vi "GetESN.vi"(9 "MEID":string, 10 "Data":string[][](array[string])=[["8986031490021881534", "460036161669975", "2A645416CB435F94", "8006A127", "460036161669975@mycdma.cn", "DB60264368A1D188", "18101891253", "A1000021A59070"], ["8986031490021881535", "460036161669976", "32FA5764D69C76BE", "80FAE4E6", "460036161669976@mycdma.cn", "B3AA1B3D2F0D5593", "18964872399", "A1000021A58D61"], ["", "", "", "", "", "", "", ""], ["", "", "", "", "", "", "", ""], ["", "", "", "", "", "", "", ""], ["", "", "", "", "", "", "", ""], ["", "", "", "", "", "", "", ""], ["", "", "", "", "", "", "", ""], ["", "", "", "", "", "", "", ""], ["", "", "", "", "", "", "", ""], ["", "各位，模块烧号主要是写五码，包括IMSI、AKEY、MEID（ESN）、AN(EVDO USER)、AAA(EVDO PWD)。", "", "", "", "", "", ""], ["", "其中ESN和MEID在模块出厂时已经写入，两者均可通过AT指令读取，但ESN不可更改。", "", "", "", "", "", ""], ["", "经询问及实际测试，上海电信绑定ESN号而广东电信未绑定，意味着上海电信五码烧录到其它模块是不可用的，但广东电信则无此限制。", "", "", "", "", "", ""], ["", "", "", "", "", "", "", ""], ["", "", "", "", "", "", "", ""], ["", "目前已确定跟上海电信合作，后续模块及卡号使用过程中，如遇到模块损坏，则意味着该卡必须销号（除非向电信申请绑定新的ESN），否则烧录到其它模块中是没用的。", "", "", "", "", "", ""]]) -> (2 "ESN":string)   [LabVIEW 2013]
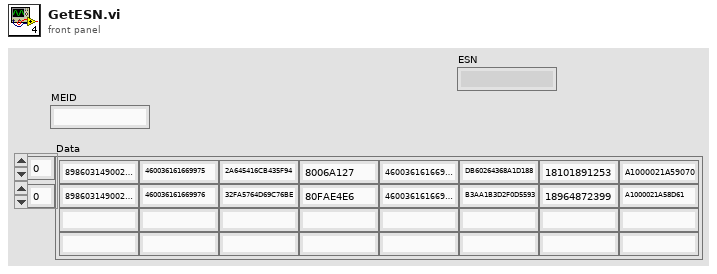
[diagram p1: front panel]
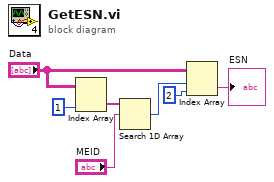
[diagram p0: block diagram]
diagram:
  n1 = Index Array(array="Data", index (col)=1 ("禁用的索引 (列)")) -> (element=w7:string[])  [unwired: 1 in]
  n2 = Search 1D Array(1D array=w7, element="MEID") -> (index of element=w2:i32)  [unwired: 1 in]
  n3 = Index Array(array="Data", index (row)=w2, index (col)=2 ("禁用的索引 (列)")) -> (element=→"ESN":string)
